vi "ExecuteTrajectory.vi"(10 "Init":bool, 11 "Trajectory":T1 {"States"."POSE"."ROTATION"."SIN" format="%13.4f"; "States"."POSE"."ROTATION"."COS" format="%13.4f"; "States"."POSE"."ROTATION"."VALUE" format="%13.4f"; "States"."POSE"."TRANSLATION"."Y" format="%14.3f"; "States"."POSE"."TRANSLATION"."X" format="%14.3f"; "TotalTImeSecs" format="%20.3f"}) -> (0 "Done":bool, 1 "LeftSpeed":dbl, 2 "RightSpeed":dbl, 3 "AtReference":bool)   [LabVIEW 2020]
uses:
  <vilib>/Rock Robotics/WPI/ThirdParty/JAS_Junk/TrajLib/TRAJECTORY.ctl
  <vilib>/Rock Robotics/WPI/ThirdParty/JAS_Junk/TrajLib/TRAJ_STATE.ctl
  <vilib>/Rock Robotics/WPI/ThirdParty/JAS_Junk/TrajLib/POSE2D.ctl
  <vilib>/Rock Robotics/WPI/ThirdParty/JAS_Junk/TrajLib/TRANSLATION2D.ctl
  <vilib>/Rock Robotics/WPI/ThirdParty/JAS_Junk/TrajLib/ROTATION2D.ctl
  <vilib>/Rock Robotics/WPI/ThirdParty/JAS_Junk/TrajLib/Conv_Feet_Meters.vi
  <vilib>/Rock Robotics/WPI/ThirdParty/JAS_Junk/TrajLib/Conv_Deg_Radians.vi
  <vilib>/Rock Robotics/WPI/ThirdParty/JAS_Junk/TrajLib/Ramsete_Execute.vi
  <vilib>/Rock Robotics/WPI/ThirdParty/JAS_Junk/TrajLib/Conv_Meters_Feet.vi
  <vilib>/Rock Robotics/WPI/ThirdParty/JAS_Junk/TrajLib/Conv_POSE_SI_Eng.vi
  <vilib>/Rock Robotics/WPI/ThirdParty/JAS_Junk/TrajLib/Ramsete_New_B_Z.vi
  <vilib>/Rock Robotics/WPI/ThirdParty/JAS_Junk/TrajLib/Ramsete_SetTolerance.vi
  <vilib>/Rock Robotics/WPI/ThirdParty/JAS_Junk/TrajLib/Pose_New.vi
  <vilib>/Rock Robotics/WPI/ThirdParty/JAS_Junk/TrajLib/Conv_AngleRadians_Heading.vi
  <vilib>/Rock Robotics/WPI/ThirdParty/JAS_Junk/TrajLib/Ramsete_SetEnabled.vi
  <vilib>/Rock Robotics/WPI/ThirdParty/JAS_Junk/TrajLib/Conv_Radians_Deg.vi
  <vilib>/Rock Robotics/WPI/ThirdParty/JAS_Junk/TrajLib/Rotation_CreateAngle.vi
  <vilib>/Rock Robotics/WPI/ThirdParty/JAS_Junk/TrajLib/Translation_Create.vi
  DriveGlobals.vi
  <vilib>/Rock Robotics/WPI/ThirdParty/JAS_Junk/TrajLib/Ramsete_Diff_DO_SI.vi
  <vilib>/Rock Robotics/WPI/ThirdParty/JAS_Junk/TrajLib/DiffWheel_Normalize.vi
  <vilib>/Rock Robotics/WPI/ThirdParty/JAS_Junk/TrajLib/Trajectory_Library.lvlib
  Autonomous/AutoGlobals.vi
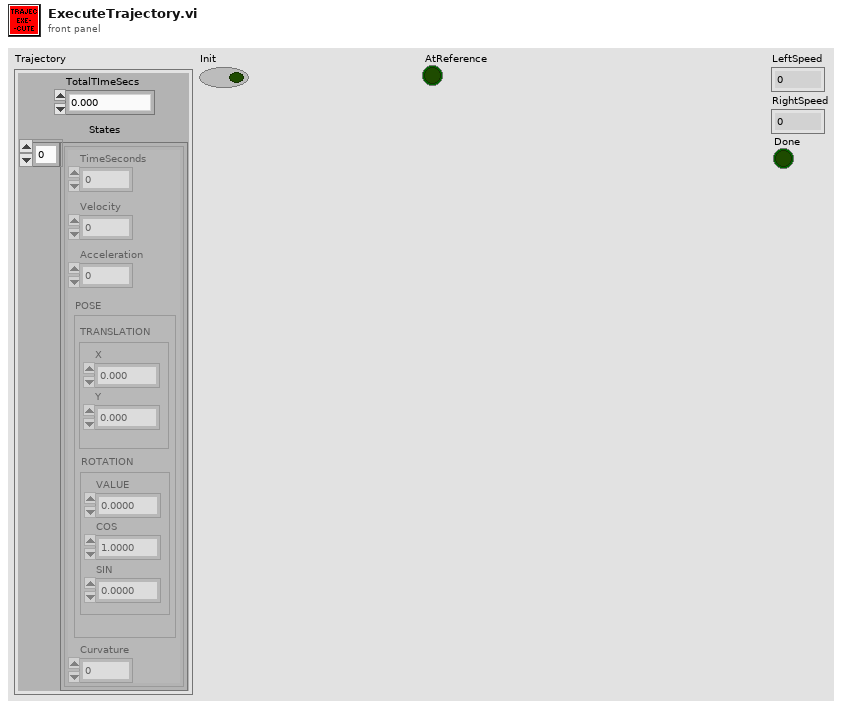
[diagram p1: front panel]
types:
  T1 = typedef "Trajectory_Library.lvlib/TRAJECTORY.ctl" = cluster{"TotalTImeSecs":dbl, "States":T2[]}
  T2 = typedef "Trajectory_Library.lvlib/TRAJ_STATE.ctl" = cluster{"TimeSeconds":dbl, "Velocity":dbl, "Acceleration":dbl, "POSE":T3, "Curvature":dbl}
  T3 = typedef "Trajectory_Library.lvlib/POSE2D.ctl" = cluster{"TRANSLATION":T4, "ROTATION":T5}
  T4 = typedef "Trajectory_Library.lvlib/TRANSLATION2D.ctl" = cluster{"X":dbl, "Y":dbl}
  T5 = typedef "Trajectory_Library.lvlib/ROTATION2D.ctl" = cluster{"VALUE":dbl, "COS":dbl, "SIN":dbl}
  T6 = typedef "Trajectory_Library.lvlib/RAMSETE_EXE_TUNING.ctl" = cluster{"B":dbl, "Zeta":dbl, "X Tolerance M":dbl, "Y Tolerance M":dbl, "Heading Tolerance RAD":dbl, "Track Width M":dbl, "Max Speed M/S":dbl}
  T7 = typedef "Trajectory_Library.lvlib/RAMSETE.ctl" = cluster{"B":dbl, "Zeta":dbl, "poseTolerance":T3, "poseError":T3, "Enabled":bool}
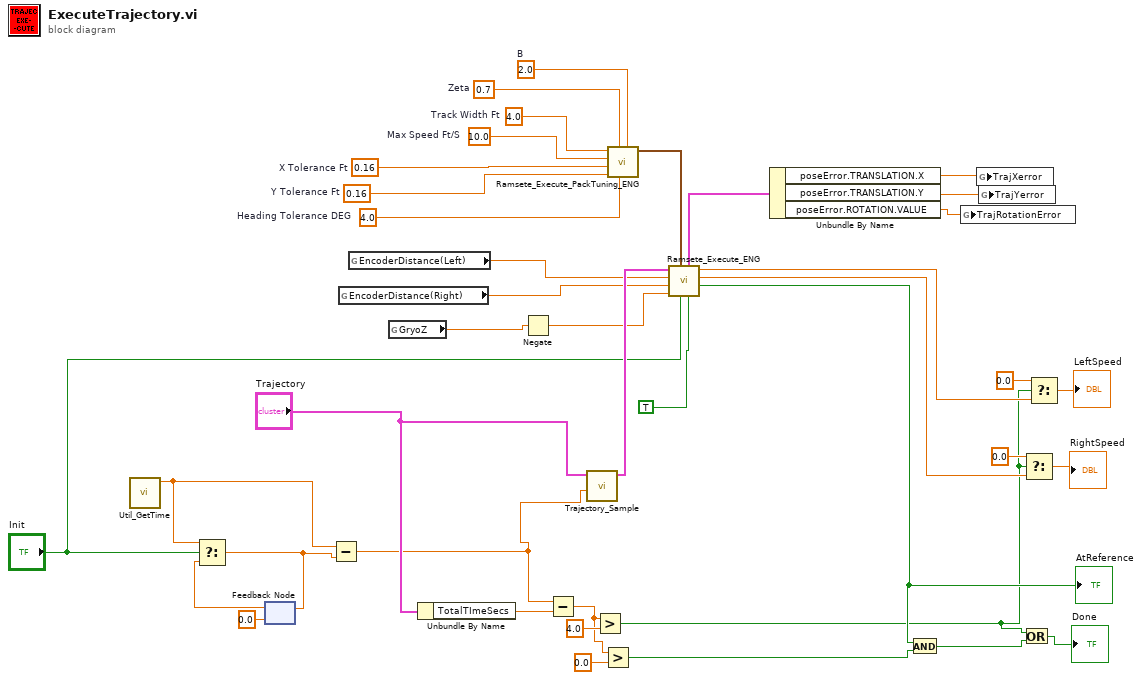
[diagram p0: block diagram]
diagram:
  w33 = 4.0  # Heading Tolerance DEG
  w34 = 0.16  # Y Tolerance Ft
  w35 = 0.16  # X Tolerance Ft
  w36 = 10.0  # Max Speed Ft/S
  w37 = 4.0  # Track Width Ft
  w38 = 0.7  # Zeta
  w39 = 2.0  # B
  n1 = call <vilib>:"Util_GetTime.vi"() -> ("FPGA_Time_Seconds"=w24:dbl)  [unwired: 10 in, 1 out]
  n2 = feedback #1(0.0) -> (w27:dbl)
  n3 = Select(t=w24, s="Init", f=w27) -> (s? t:f=w26:dbl)
  n4 = feedback-in #1(w26) -> ()
  n5 = Subtract(x=w24, y=w26) -> (x-y=w29:dbl)
  n6 = global read "DriveGlobals.vi" "EncoderDistance(Right)"() -> (w17:dbl)
  n7 = global read "DriveGlobals.vi" "EncoderDistance(Left)"() -> (w16:dbl)
  n8 = global read "DriveGlobals.vi" "GryoZ"() -> (w6:dbl)
  n9 = Unbundle By Name("Trajectory") -> ("TotalTImeSecs"=w30:dbl)
  n10 = Negate(x=w6) -> (-x=w5:dbl)
  n11 = Subtract(x=w29, y=w30) -> (x-y=w13:dbl)
  n12 = call <vilib>:"Trajectory_Sample.vi"("Time"=w29, "InputTRAJECTORY"="Trajectory") -> ("OutputTRAJ_STATE"=w32:T2)  [unwired: 9 in]
  n13 = Greater?(x=w13, y=4.0) -> (0:w8:bool)
  n14 = Greater?(x=w13, y=0.0) -> (0:w10:bool)
  n15 = call <vilib>:"Ramsete_Execute_PackTuning_ENG.vi"("B"=w39, "Heading Tolerance DEG"=w33, "Zeta"=w38, "Y Tolerance Ft"=w34, "X Tolerance Ft"=w35, "Max Speed Ft/S"=w36, "Track Width Ft"=w37) -> ("RAMSETE_EXE_TUNING"=w40:T6)  [unwired: 4 in]
  n16 = call <vilib>:"Ramsete_Execute_ENG.vi"("Enabled"=TRUE, "Reset"="Init", "RAMSETE_EXE_TUNING"=w40, "Gyro-Deg\n(Inc counterclockwise)"=w5, "RightDist-Ft"=w17, "LeftDist-Ft"=w16, "TRAJ_STATE  SI"=w32) -> ("AtReference"=w11:bool, "Right Speed Dmd Ft/S"=w14:dbl, "Left Speed Dmd Ft/S"=w15:dbl, "outRAMSETE"=w4:T7)  [unwired: 1 out]
  "AtReference" <- w11
  n17 = Unbundle By Name(w4) -> ("poseError.TRANSLATION.X"=w3:dbl, "poseError.TRANSLATION.Y"=w1:dbl, "poseError.ROTATION.VALUE"=w2:dbl)
  n18 = And(x=w11, y=w10) -> (x .and. y?=w7:bool)
  n19 = global write "AutoGlobals.vi" "TrajRotationError"(w2) -> ()
  n20 = global write "AutoGlobals.vi" "TrajXerror"(w3) -> ()
  n21 = global write "AutoGlobals.vi" "TrajYerror"(w1) -> ()
  n22 = Or(x=w8, y=w7) -> (x .or. y?=→"Done":bool)
  n23 = Select(t=0.0, s=w8, f=w14) -> (s? t:f=→"RightSpeed":dbl)
  n24 = Select(t=0.0, s=w8, f=w15) -> (s? t:f=→"LeftSpeed":dbl)
